vi "FuncImg-Init intensity zoom ctrl.vi"   [LabVIEW 2013]
uses:
  Global variables/gl_Functional Imaging-Global variables.vi
types:
  T1 = typedef "Functional Imging UI Refs.ctl" = cluster{"Menu ref":refnum<k9>, "Image control":refnum<vi>, "VI ref":refnum<vi>, "XGrapher":refnum<vi>, "Smoothing":refnum<vi>, "POI Averaging":refnum<vi>, "Normalize":refnum<vi>, "POI data points in each trial":refnum<vi>, "Channel":refnum<vi>, "Experiment data folder path":refnum<vi>, "[ROI vis]":refnum<vi>, "[Groups] visbl":T2, "Group Name":refnum<vi>, "POI index":refnum<vi>, "Trial No.":refnum<vi>, "Intensity Zoom":refnum<vi>, "Trial Cursor Enabled":refnum<vi>, "Number of Trials (ind 1)":refnum<vi>, "Number of Trials (ind 2)":refnum<vi>, "MiniScans Available":refnum<vi>, "POI Available":refnum<vi>, "Defer graph updates":refnum<vi>, "Waveform selector":refnum<vi>, "#of selected POI":refnum<vi>, "#of selected MiniScans":refnum<vi>, "#of selected groups":refnum<vi>, "Max Z-Projection":refnum<vi>, "Z-Plane Selector":refnum<vi>, "Index of miniscan point to visualise":refnum<vi>, "ROI vis. mode":refnum<vi>, "Total # of points":refnum<vi>, "Index of group clicked on":refnum<vi>, "Pane 1":refnum<vi>, "Pane 2":refnum<vi>, "Pane 3":refnum<vi>, "Pane 4":refnum<vi>, "Pane 5":refnum<vi>, "Pane 6":refnum<vi>, "Deselect all ROI":refnum<vi>, "Deselect all groups":refnum<vi>}
  T2 = typedef "Groups array referecne.ctl" = refnum<vi>
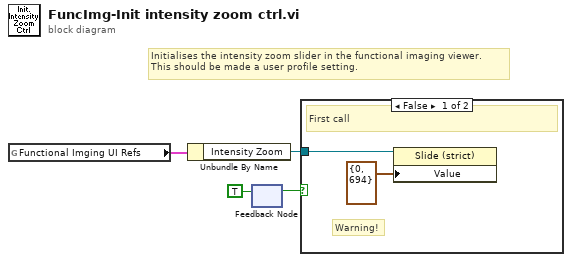
[diagram p0: block diagram]
diagram:
  # "Initialises the intensity zoom slider in the functional imaging viewer.\nThis should be made a user profile setting."
  n1 = global read "gl_Functional Imaging-Global variables.vi" "Functional Imging UI Refs"() -> (w2:T1)
  n2 = Unbundle By Name(w2) -> ("Intensity Zoom"=w1:refnum<vi>)
  n3 = feedback #1() -> (w4:bool)  [unwired: 1 in]
  n4 = feedback-in #1(TRUE) -> ()
  n5 = case shown="False" w4 {
    tunnel: w1 -> [w5 _]
    frame False {
      # "Warning!"
      # "First call"
      n6 = property class="Slide (strict)"(reference=w5, "Value"=cluster{u16, u16} {0, 694} ("LUT")) -> ()  [unwired: 1 in, 2 out]
    }
    frame True {
    }
  }
